vi "mod_Generate Profile Definition.vi"(6 "on level":dbl format="%.2f", 7 "burst length":dbl=146.0 format="%.1f", 8 "ramp start level":dbl format="%.2f", 9 "off level":dbl=-inf format="%.2f", 10 "off time":dbl=5.0 format="%.1f", 11 "ramp time":dbl=5.0 format="%.1f") -> (3 "profile definition":cluster{"time":dbl, "power (dB)":dbl}[](array[cluster]) {"power (dB)" format="%.2f"; "time" format="%.2f"})   [LabVIEW 2020, in "niDMT.lvlib"]
uses:
  <vilib>/addons/Modulation/niDMT.lvlib
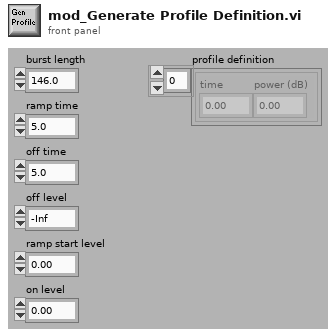
[diagram p1: front panel]
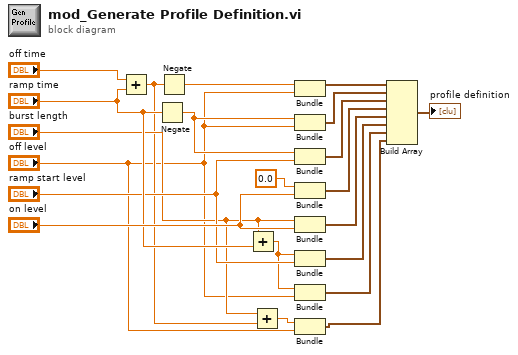
[diagram p0: block diagram]
diagram:
  n1 = Add(x="off time", y="ramp time") -> (x+y=w11:dbl)
  n2 = Negate(x="ramp time") -> (-x=w19:dbl)
  n3 = Negate(x=w11) -> (-x=w20:dbl)
  n4 = Add(x="burst length", y="ramp time") -> (x+y=w14:dbl)
  n5 = Add(x="burst length", y=w11) -> (x+y=w13:dbl)
  n6 = Bundle(w20, "off level"="off level") -> (w9:cluster{dbl, "off level":dbl})  [unwired: 1 out]
  n7 = Bundle(w19, "off level"="off level") -> (w8:cluster{dbl, "off level":dbl})  [unwired: 1 out]
  n8 = Bundle(w19, "ramp start level"="ramp start level") -> (w7:cluster{dbl, "ramp start level":dbl})  [unwired: 1 out]
  n9 = Bundle(0.0, "on level"="on level") -> (w6:cluster{dbl, "on level":dbl})  [unwired: 1 out]
  n10 = Bundle("burst length"="burst length", "on level"="on level") -> (w5:cluster{"burst length":dbl, "on level":dbl})  [unwired: 1 out]
  n11 = Bundle(w14, "ramp start level"="ramp start level") -> (w4:cluster{dbl, "ramp start level":dbl})  [unwired: 1 out]
  n12 = Bundle(w14, "off level"="off level") -> (w3:cluster{dbl, "off level":dbl})  [unwired: 1 out]
  n13 = Bundle(w13, "off level"="off level") -> (w2:cluster{dbl, "off level":dbl})  [unwired: 1 out]
  n14 = Build Array(w9, w8, w7, w6, w5, w4, w3, w2) -> (→"profile definition":cluster{"burst length":dbl, "off level":dbl}[])
